vi "SeCrTs-RT_Main.vi"() -> ()   [LabVIEW 2022 SP3]
uses:
  <vilib>/Platform/TimedLoop/XDataNode/timing_clust.ctl
  <vilib>/Platform/TimedLoop/XDataNode/nitl_modes.ctl
  <vilib>/Platform/TimedLoop/XDataNode/wakeup.ctl
  RT Support/SeCrTs-RT_Global_R.vi
  <vilib>/platform/TimedLoop/XDataNode/XDataNode.xnode
  <vilib>/Platform/TimedLoop/XDataNode/XDNodeRunTimeDep.lvlib
panel:
  out "CDT":dbl
  # "RT main"
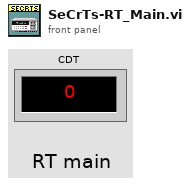
[diagram p1: front panel]
types:
  T1 = enum16{"Init", "Read 'All'", "Read 'n'", "Read '1'", "Write '1'", "Write 'n'", "Write 'All'"}
  T2 = cluster{"Device List":cluster{"AO Cards":tag[], "AI Cards":tag[], "DI Cards":tag[], "DO Cards":tag[]}, "Channel List":cluster{"AI Channel list":tag[], "AO Channel list":tag[], "DO Channel list ":tag[], "DI Channel list":tag[]}}
  T3 = cluster{"Drive Control":cluster{"En_Drive_A":bool, "En_Drive_L":bool, "Exit_Drive_A":bool, "Exit_Drive_L":bool}, "Drive_ATF Control":cluster{"S.Freq":dbl, "Ramp up Time":dbl, "Ramp down Time":dbl, "Drive Speed":dbl, "Drive condition":dbl}, "Drive_LOX Control":cluster{"S.Freq":dbl, "Ramp up Time":dbl, "Ramp down Time":dbl, "Drive Speed":dbl, "Drive condition":dbl}, "Aconnection ID":refnum<k5>, "Lconnection ID":refnum<k5>, "Loop Control":cluster{"Start DAQ":bool, "Stop DAQ":bool, "RT Stop":bool, "RT Exit":bool, "Start Seq":bool}}
  T4 = cluster{"AO Cards":tag[], "AI Cards":tag[], "DI Cards":tag[], "DO Cards":tag[]}
  T5 = cluster{"AI Channel list":tag[], "AO Channel list":tag[], "DO Channel list ":tag[], "DI Channel list":tag[]}
  T6 = typedef "SeCrTs-Data FIFO.ctl" = cluster{"Control":cluster{"AI_V_Data":refnum<queue>, "AI_C_Data":refnum<queue>, "AO_Data":refnum<queue>, "DO_Data":refnum<queue>, "DI_Data":refnum<queue>, "ACC_Data":refnum<queue>, "TC_Data":refnum<queue>, "Drive_A_C":refnum<queue>, "Drive_A_D":refnum<queue>, "Drive_L_C":refnum<queue>, "Drive_L_D":refnum<queue>}, "Display":cluster{"AI_V_Data D":refnum<queue>, "AI_C_Data D":refnum<queue>, "AO_Data D":refnum<queue>, "DO_Data D":refnum<queue>, "DI_Data D":refnum<queue>, "ACC_Data D":refnum<queue>, "TC_Data D":refnum<queue>, "Drive_A_C D":refnum<queue>, "Drive_A_D D":refnum<queue>, "Drive_L_C D":refnum<queue>, "Drive_L_D D":refnum<queue>}, "RD":cluster{"AI_V_Data RD":refnum<queue>, "AI_C_Data RD":refnum<queue>, "AO_Data RD":refnum<queue>, "DO_Data RD":refnum<queue>, "DI_Data RD":refnum<queue>, "ACC_Data RD":refnum<queue>, "TC_Data RD":refnum<queue>, "Drive_A_C RD":refnum<queue>, "Drive_A_D RD":refnum<queue>, "Drive_L_C RD":refnum<queue>, "Drive_L_D RD":refnum<queue>}}
  T7 = typedef "XDNodeRunTimeDep.lvlib/timing_clust.ctl" = cluster{"Expected End [f-1]":u64, "Actual End [f-1]":u64, "Finished Late? [f-1]":bool, "Expected End [i-1]":u64, "Actual End [i-1]":u64, "Finished Late? [i-1]":bool, "Expected Start [i]":u64, "Actual Start [i]":u64, "Expected Start [f]":u64, "Actual Start [f]":u64, "Source Name":string, "Structure Name":string, "Period":i64, "Deadline":i64, "Offset":i64, "Start":i64, "Priority":i32, "Timeout":i32, "Mode":T8, "Wakeup Reason":T9, "Error":errorcluster, "Source Type":string, "Secondary Source Type":string, "Global End Time":u64, "Global Start Time":u64, "Frame Duration":u64, "Iteration Duration":u64, "Assigned CPU":i32, "I/O Scan Engine Mode":u32}
  T8 = typedef "XDNodeRunTimeDep.lvlib/nitl_modes.ctl" = enum32{"No Change", "Process missed periods, maintain original phase", "Discard missed periods, maintain original phase", "Process missed periods, ignore original phase", "Discard missed periods, ignore original phase"}
  T9 = typedef "XDNodeRunTimeDep.lvlib/wakeup.ctl" = enum32{"Normal", "Aborted", "Asynchronous wakeup", "Timing source error", "Timed loop error", "Timeout"}
  T10 = cluster{cluster{"Sr. No.":string, "Time CDT":string, "Component ID":string, "Data Type":string, "Condition":string, "Range/Position":string, "No of Samples for Pass":string, "Event Duration":string, "Continuous /Cumulative":string, "Expected Delay":string, "Failure case Seq":string, "Current Sequence":string}[]}[]
  T11 = cluster{"AO config":cluster{"Channel_Name":string, "Channel_Number":string, "Default_Value":dbl, "Units":string}[], "AI config":cluster{"Channel_Name":string, "Channel_Number":string, "Pre_Scale_min":dbl, "Pre_Scale_max":dbl, "Sensor_min":dbl, "Sensor_max":dbl, "Units":string}[], "DI config":cluster{"Channel_Name":string, "Channel_Number":string, "Default_Value":bool, "DI invert?":bool}[], "DO config":cluster{"Channel_Name":string, "Channel_Number":string, "Default_Value":bool, "DO invert?":bool}[], "TC config":cluster{"Channel_Name":string, "Channel_Number":string, "Pre_Scale_min":dbl, "Pre_Scale_max":dbl, "units":i32, " type":i32}[], "ACC config":cluster{"Channel_Name":string, "Channel_Number":string, "Pre_Scale_min":dbl, "Pre_Scale_max":dbl, "Terminal configuration":i32, "Sensitivity":dbl, "Sensitivity units":i32}[], "SG config":cluster{"Channel_Name":string, "Channel_Number":string, "Pre_Scale_min":dbl, "Pre_Scale_max":dbl}[], "Strain Gauge Settings":cluster{"poisson ratio":dbl, "nominal gage resistance":dbl, "gage factor":dbl}, "Bridge Settings":cluster{"voltage excitation value":dbl, "voltage excitation source":i32, "initial bridge voltage":dbl, "lead wire resistance":dbl, "strain configuration":i32}, "Sample Rate":cluster{"AI Sample Rate":dbl[], "AO Sample Rate":dbl[], "DI Sample Rate":dbl[], "TC Sample Rate":dbl[], "DO Sample Rate":dbl[], "SG Sample Rate":dbl[], "ACC Sample Rate":dbl[]}}
  T12 = enum16{"Init", "Read", "Write 'All'", "Write 'n'", "Write Safe Value", "Write Start Time", "Overwrite Pattern", "Overwrite Pattern with Start", "Append Pattern", "Start Pattern Mode", "Abort Pattern Mode", "Read 1"}
  T13 = cluster{"S.Freq":dbl, "Ramp up Time":dbl, "Ramp down Time":dbl, "Drive Speed":dbl, "Drive condition":dbl}
  T14 = cluster{"Start DAQ":bool, "Stop DAQ":bool, "RT Stop":bool, "RT Exit":bool, "Start Seq":bool}
  T15 = cluster{"En_Drive_A":bool, "En_Drive_L":bool, "Exit_Drive_A":bool, "Exit_Drive_L":bool}
  T16 = cluster{"Manual HOLD":bool, "Automatic Hold AI":bool, "Abort":bool, "Automatic Hold DI":bool}
  T17 = cluster{"Channel_Name":string, "Channel_Number":string, "Default_Value":bool, "DO invert?":bool}[]
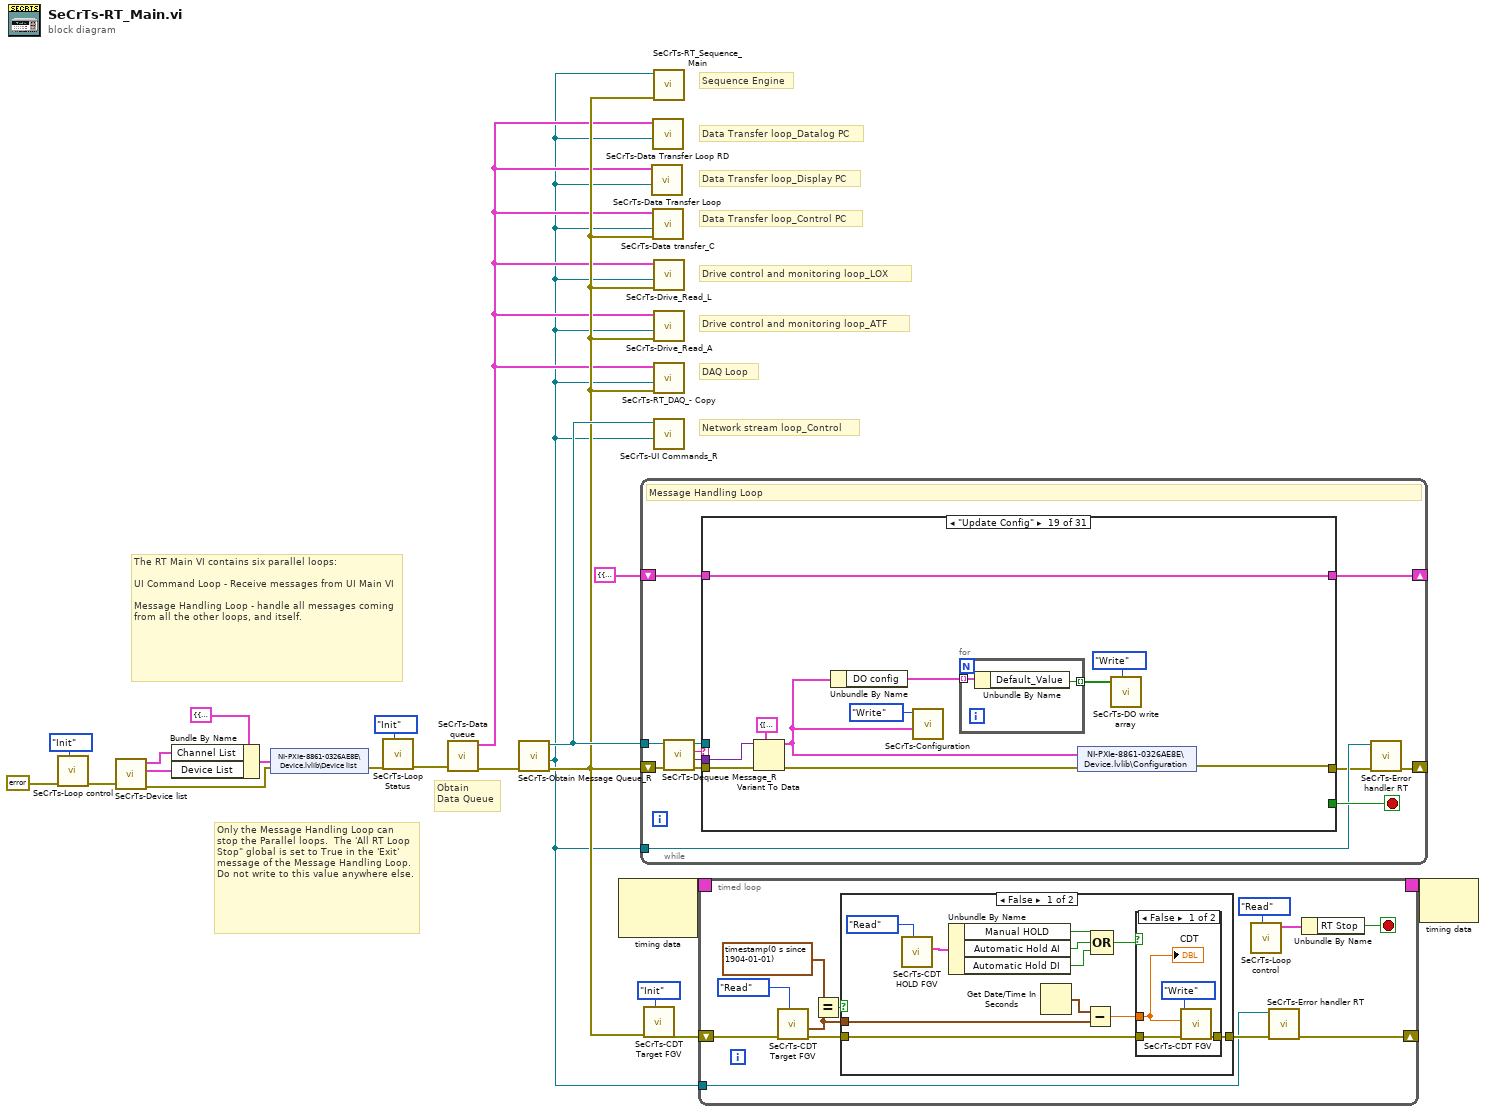
[diagram p0: block diagram]
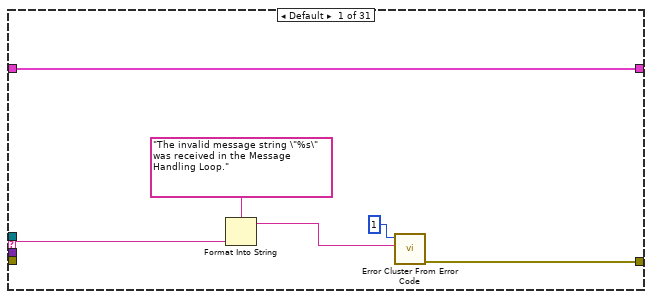
[diagram p4: hidden frame]
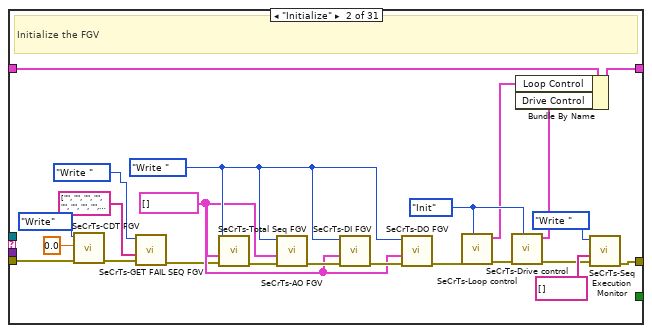
[diagram p5: hidden frame]
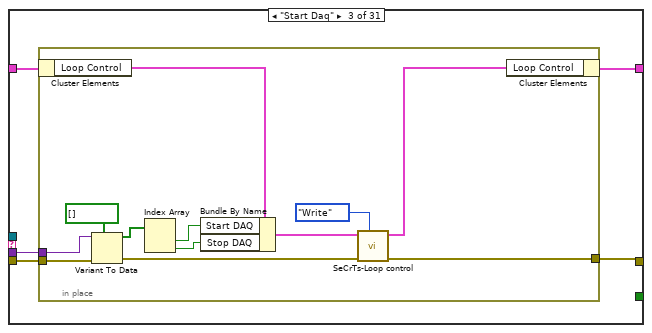
[diagram p6: hidden frame]
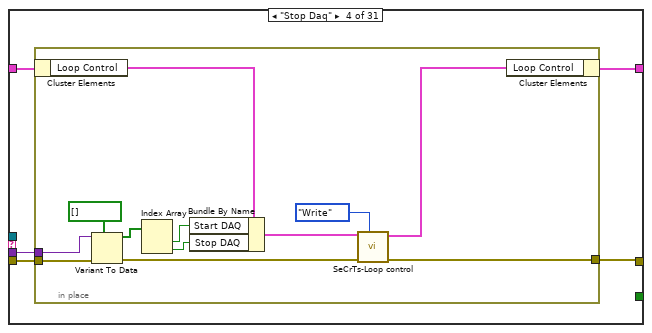
[diagram p7: hidden frame]
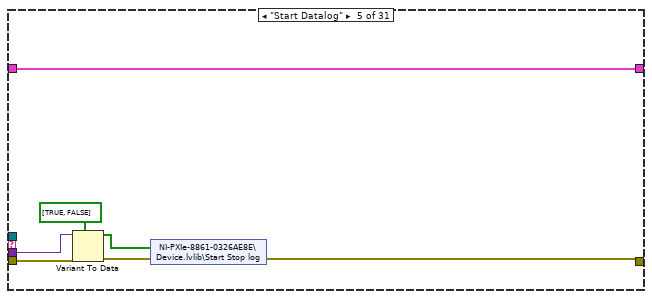
[diagram p8: hidden frame]
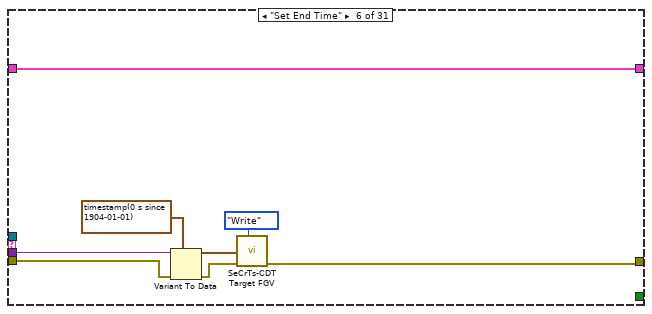
[diagram p9: hidden frame]
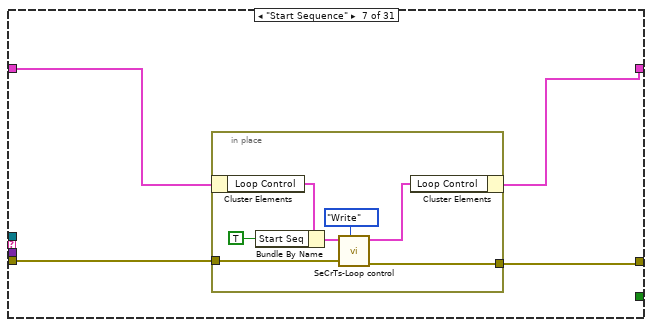
[diagram p10: hidden frame]
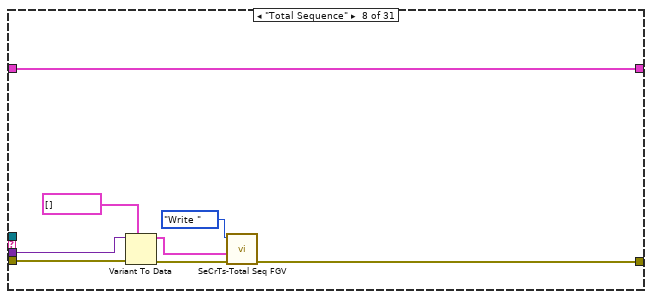
[diagram p11: hidden frame]
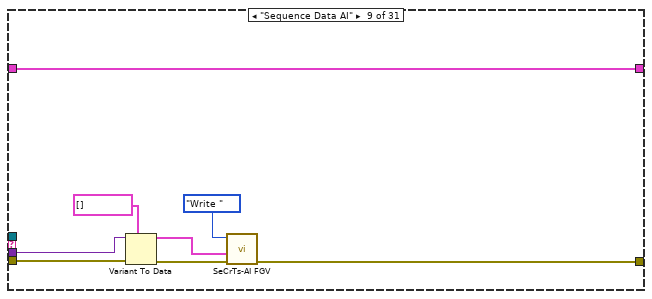
[diagram p12: hidden frame]
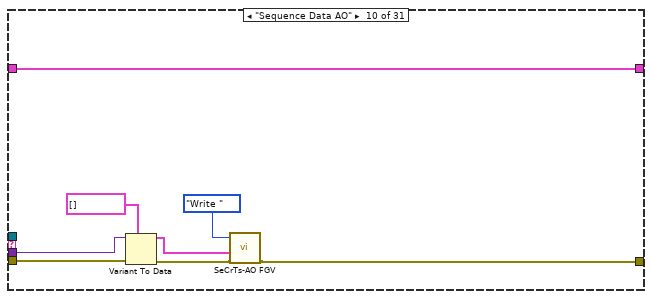
[diagram p13: hidden frame]
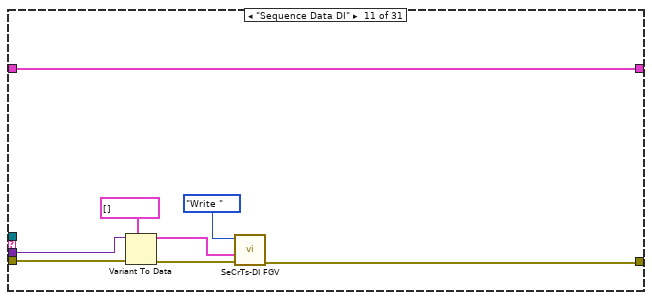
[diagram p14: hidden frame]
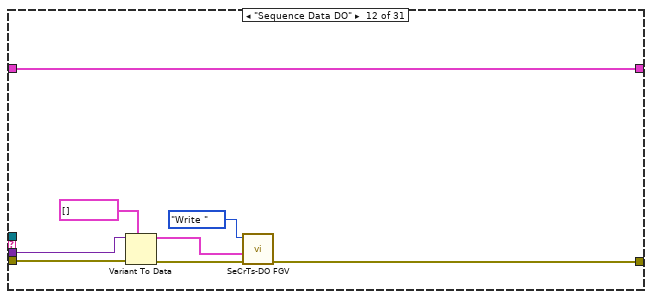
[diagram p15: hidden frame]
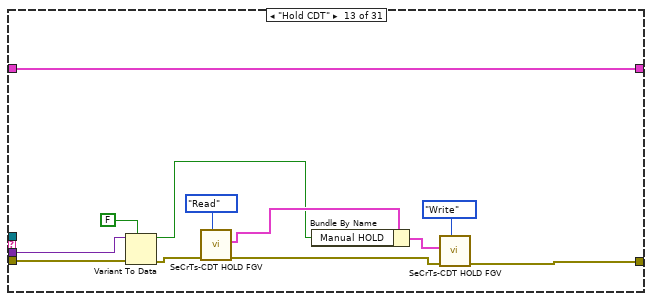
[diagram p16: hidden frame]
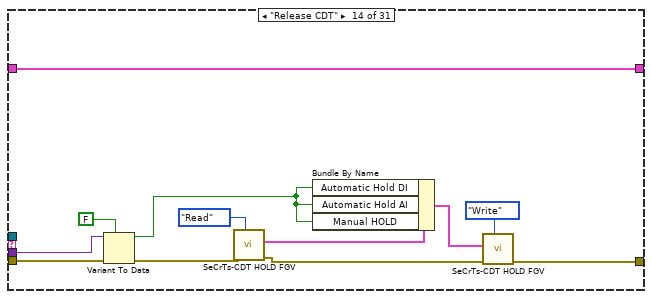
[diagram p17: hidden frame]
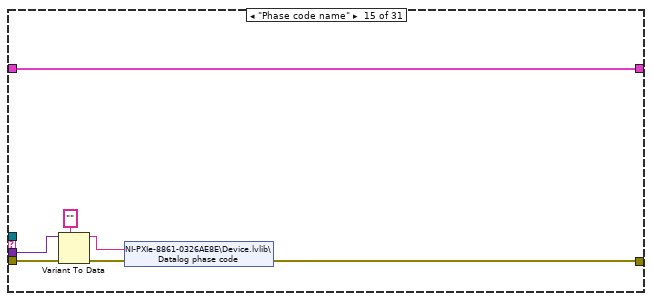
[diagram p18: hidden frame]
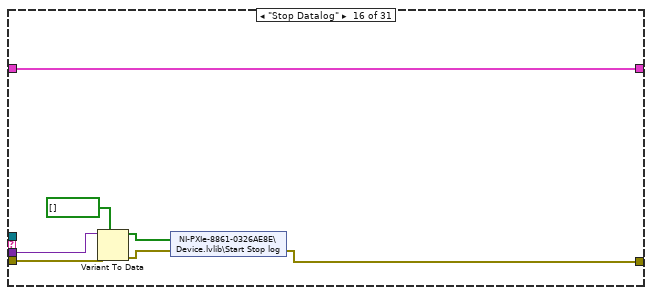
[diagram p19: hidden frame]
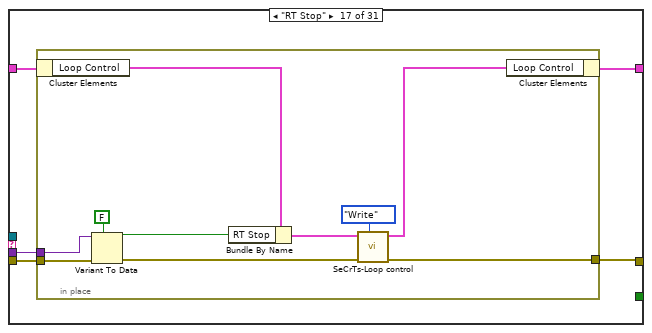
[diagram p20: hidden frame]
diagram:
  # "Sequence Engine"
  # "Data Transfer loop_Display PC"
  # "Data Transfer loop_Control PC"
  # "Drive control and monitoring loop_LOX"
  # "Drive control and monitoring loop_ATF"
  # "DAQ Loop"
  # "Data Transfer loop_Datalog PC"
  # "Obtain\nData Queue"
  # "Network stream loop_Control"
  # "The RT Main VI contains six parallel loops:\n\nUI Command Loop - Receive messages from UI Main VI\n\nMessage Handling Loop - handle all messages coming from all the other loops, and itself."
  # "Only the Message Handling Loop can stop the Parallel loops.  The 'All RT Loop Stop\" global is set to True in the 'Exit' message of the Message Handling Loop.  Do not write to this value anywhere else."
  n1 = call "SeCrTs-Loop control.vi"("Action"=enum16{"Init", "Write", "Read"}."Init", "error in (no error)"=errorcluster {"status"=FALSE, "code"=0, "source"=""} ("error constant")) -> ("error Out"=w6:errorcluster)  [unwired: 8 in, 1 out]
  n2 = call "SeCrTs-Device list.vi"("error in (no error)"=w6) -> ("error out"=w12:errorcluster, "Device List"=w14:T4, "Channel List"=w15:T5)  [unwired: 8 in]
  n3 = Bundle By Name(cluster=T2 {"Device List"={"AO Cards"=[], "AI Cards"=[], "DI Cards"=[], "DO Cards"=[]}, "Channel List"={"AI Channel list"=[], "AO Channel list"=[], "DO Channel list "=[], "DI Channel list"=[]}}, "Channel List"=w15, "Device List"=w14) -> (w13:T2)
  n4 = shared-variable "NI-PXIe-8861-0326AE8E\\Device.lvlib\\Device list"(w13, error in=w12) -> (error out=w10:errorcluster)
  n5 = call "SeCrTs-Loop Status.vi"("Option"=T1."Init", "error in (no error)"=w10) -> ("error out"=w9:errorcluster)  [unwired: 7 in, 2 out]
  n6 = call "SeCrTs-Data queue.vi"("error in"=w9) -> ("Data FIFO Ref"=w17:T6, "error out"=w18:errorcluster)  [unwired: 8 in]
  n7 = call "SeCrTs-Obtain Message Queue_R.vi"("error in (no error)"=w18) -> ("error out"=w20:errorcluster, "queue out"=w5:refnum<queue>, "Message Queue"=w21:refnum<queue>)  [unwired: 8 in]
  n8 = node-c288() -> (w4:T7)  [unwired: 2 in]
  n9 = while {
    shift-right: [w22] -> _
    shift-left: w20 -> [w33]
    tunnel: w21 -> [w31]
    shift-right: [w25] -> _
    shift-left: T3 {"Drive Control"={"En_Drive_A"=FALSE, "En_Drive_L"=FALSE, "Exit_Drive_A"=FALSE, "Exit_Drive_L"=FALSE}, "Drive_ATF Control"={"S.Freq"=0.0, "Ramp up Time"=0.0, "Ramp down Time"=0.0, "Drive Speed"=0.0, "Drive condition"=0.0}, "Drive_LOX Control"={"S.Freq"=0.0, "Ramp up Time"=0.0, "Ramp down Time"=0.0, "Drive Speed"=0.0, "Drive condition"=0.0}, "Aconnection ID"=refnum, "Lconnection ID"=refnum, "Loop Control"={"Start DAQ"=FALSE, "Stop DAQ"=FALSE, "RT Stop"=FALSE, "RT Exit"=FALSE, "Start Seq"=FALSE}} -> [w26]
    tunnel: w5 -> [w24]
    stop <- w27 stop-if-true
    # "Message Handling Loop"
    n10 = call "SeCrTs-Dequeue Message_R.vi"("error in (no error)"=w33, "Message Queue"=w31) -> ("error out"=w29:errorcluster, "Message Data"=w30:variant, "Message"=w32:string, "dup Message Queue"=w28:refnum<queue>)  [unwired: 6 in]
    n11 = case shown="\"Update Config\"" w32 {
      selector: w32 -> [w35 _ _ _ _ _ _ _ _ _ _ _ _ _ _ _ _ _ _ _ _ _ _ _ _ _ _ _ _ _ _]
      tunnel: w28 -> [_ _ _ _ _ _ _ _ _ _ _ _ _ _ _ _ _ _ _ _ _ _ _ _ _ _ _ _ _ _ w365]
      tunnel: w30 -> [_ _ w65 w82 w101 w110 _ w126 w134 w144 w152 w160 w172 w181 w191 w196 w203 _ w224 _ w246 _ w253 w267 w282 w297 w312 w336 _ _ w363]
      tunnel: w29 -> [_ w55 w67 w84 w102 w109 w113 w128 w136 w145 w153 w161 w173 w184 w192 w197 w205 _ w225 w231 w247 _ w254 w268 w283 w298 w313 w337 _ _ w364]
      tunnel: [w34 w41 w66 w83 w97 w105 w114 w124 w133 w142 w150 w159 w169 w183 w187 w194 w204 _ w217 w230 w243 _ w252 w266 w281 w296 w311 w335 _ _ w362] -> w23
      tunnel: [_ _ _ _ _ _ _ _ _ _ _ _ _ _ _ _ _ _ _ _ _ _ _ _ _ _ _ _ _ _ w361] -> w27
      tunnel: w26 -> [w39 w58 w64 w81 w103 w111 w115 w130 w138 w146 w154 w162 w174 w186 w193 w200 w202 w216 w227 w233 w248 w249 w251 w265 w280 w295 w310 w334 w357 w358 w360]
      tunnel: [w39 w57 w63 w80 w103 w111 w112 w130 w138 w146 w154 w162 w174 w186 w193 w200 w201 w216 w227 w232 w248 w249 w250 _ w279 w294 w309 w333 w357 w358 w359] -> w25
      frame Default {
        n12 = Format Into String(format string="The invalid message string \"%s\" was received in the Message Handling Loop." ("Unknown Message Error Text"), w35) -> (resulting string=w36:string)  [unwired: 2 in, 1 out]
        n13 = call <vilib>:"Error Cluster From Error Code.vi"("error message (\"\")"=w36, "error code (0)"=1) -> ("error out"=w34:errorcluster)  [unwired: 7 in]
      }
      frame "Initialize" {
        w48 = T10 [] ("Array")
        w56 = enum16{"Read", "Write "}."Write " ("Enum")
        w61 = enum16{"Init", "Write", "Read"}."Init" ("Action")
        # "Initialize the FGV"
        n14 = call "SeCrTs-CDT FGV.vi"("error in (no error)"=w55, "CDT"=0.0, "Write/Read"=enum16{"Write", "Read"}."Write") -> ("error Out"=w43:errorcluster)  [unwired: 7 in, 1 out]
        n15 = call "SeCrTs-GET FAIL SEQ FGV.vi"("error in"=w43, "Failure \ncase Seq"=string[] ["", "", "", "", "", "", "", "", "", ""] ("Failure \ncase Seq"), "Enum"=enum16{"Read", "Write "}."Write ") -> ("error out"=w42:errorcluster)  [unwired: 7 in, 1 out]
        n16 = call "SeCrTs-Total Seq FGV.vi"("error in"=w42, "Total Seq  IN"=w48, "Enum"=w56) -> ("error out"=w54:errorcluster)  [unwired: 7 in, 1 out]
        n17 = call "SeCrTs-AO FGV.vi"("error in"=w54, "AO Seq  IN"=w48, "Enum"=w56) -> ("error out"=w53:errorcluster)  [unwired: 7 in, 1 out]
        n18 = call "SeCrTs-DI FGV.vi"("error in"=w53, "DI Seq  IN"=w48, "Enum"=w56) -> ("error out"=w52:errorcluster)  [unwired: 7 in, 1 out]
        n19 = call "SeCrTs-DO FGV.vi"("error in"=w52, "DO Seq  IN"=w48, "Enum"=w56) -> ("error out"=w51:errorcluster)  [unwired: 7 in, 1 out]
        n20 = call "SeCrTs-Loop control.vi"("Action"=w61, "error in (no error)"=w51) -> ("error Out"=w62:errorcluster, "Loop Control out"=w60:T14)  [unwired: 8 in]
        n21 = call "SeCrTs-Drive control.vi"("Action"=w61, "error in"=w62) -> ("error Out"=w40:errorcluster, "Loop Control Out"=w59:T15)  [unwired: 8 in]
        n22 = Bundle By Name(cluster=w58, "Loop Control"=w60, "Drive Control"=w59) -> (w57:T3)
        n23 = call "SeCrTs-Seq Execution Monitor.vi"("error in"=w40, "Seq Monitor"=string[] [], "Enum"=enum16{"Read", "Write "}."Write ") -> ("error out"=w41:errorcluster)  [unwired: 7 in, 1 out]
      }
      frame "Start Daq" {
        n24 = in-place {
          in-place-border: w67 -> [w78]
          in-place-border: [w75] -> w66
          in-place-border: w65 -> [w74]
          n25 = in-place-cluster #1(w64) -> ("Loop Control"=w73:T14)
          n26 = Variant To Data(error in=w78, type=bool[] [], Variant=w74) -> (data=w70:bool[], error out=w76:errorcluster)
          n27 = Index Array(array=w70) -> (element #1=w69:bool, element #2=w68:bool)  [unwired: 2 in]
          n28 = Bundle By Name(cluster=w73, "Start DAQ"=w69, "Stop DAQ"=w68) -> (w72:T14)
          n29 = call "SeCrTs-Loop control.vi"("Action"=enum16{"Init", "Write", "Read"}."Write", "error in (no error)"=w76, "Loop Control In"=w72) -> ("error Out"=w75:errorcluster, "Loop Control out"=w71:T14)  [unwired: 7 in]
          n30 = in-place-cluster #1("Loop Control"=w71) -> (w63:T3)
        }
      }
      frame "Stop Daq" {
        n31 = in-place {
          in-place-border: w84 -> [w95]
          in-place-border: [w92] -> w83
          in-place-border: w82 -> [w91]
          n32 = in-place-cluster #2(w81) -> ("Loop Control"=w90:T14)
          n33 = Variant To Data(error in=w95, type=bool[] [], Variant=w91) -> (data=w87:bool[], error out=w93:errorcluster)
          n34 = Index Array(array=w87) -> (element #1=w86:bool, element #2=w85:bool)  [unwired: 2 in]
          n35 = Bundle By Name(cluster=w90, "Start DAQ"=w86, "Stop DAQ"=w85) -> (w89:T14)
          n36 = call "SeCrTs-Loop control.vi"("Action"=enum16{"Init", "Write", "Read"}."Write", "error in (no error)"=w93, "Loop Control In"=w89) -> ("error Out"=w92:errorcluster, "Loop Control out"=w88:T14)  [unwired: 7 in]
          n37 = in-place-cluster #2("Loop Control"=w88) -> (w80:T3)
        }
      }
      frame "Start Datalog" {
        n38 = Variant To Data(error in=w102, type=bool[] [TRUE, FALSE] ("Start Stop log"), Variant=w101) -> (data=w99:bool[], error out=w98:errorcluster)
        n39 = shared-variable "NI-PXIe-8861-0326AE8E\\Device.lvlib\\Start Stop log"(w99, error in=w98) -> (error out=w97:errorcluster)
      }
      frame "Set End Time" {
        n40 = Variant To Data(error in=w109, type=timestamp(0 s since 1904-01-01) ("current time"), Variant=w110) -> (data=w107:timestamp, error out=w106:errorcluster)
        n41 = call "SeCrTs-CDT Target FGV.vi"("Enum"=enum16{"Write", "Read", "Init"}."Write", "error in"=w106, "Time Stamp"=w107) -> ("error out"=w105:errorcluster)  [unwired: 7 in, 1 out]
      }
      frame "Start Sequence" {
        n42 = in-place {
          in-place-border: w113 -> [w117]
          in-place-border: [w116] -> w114
          n43 = in-place-cluster #3(w115) -> ("Loop Control"=w122:T14)
          n44 = Bundle By Name(cluster=w122, "Start Seq"=TRUE ("Start DAQ")) -> (w119:T14)
          n45 = call "SeCrTs-Loop control.vi"("Action"=enum16{"Init", "Write", "Read"}."Write", "error in (no error)"=w117, "Loop Control In"=w119) -> ("error Out"=w116:errorcluster, "Loop Control out"=w118:T14)  [unwired: 7 in]
          n46 = in-place-cluster #3("Loop Control"=w118) -> (w112:T3)
        }
      }
      frame "Total Sequence" {
        n47 = Variant To Data(error in=w128, type=T10 [] ("Array"), Variant=w126) -> (data=w125:T10, error out=w127:errorcluster)
        n48 = call "SeCrTs-Total Seq FGV.vi"("error in"=w127, "Total Seq  IN"=w125, "Enum"=enum16{"Read", "Write "}."Write ") -> ("error out"=w124:errorcluster)  [unwired: 7 in, 1 out]
      }
      frame "Sequence Data AI" {
        n49 = Variant To Data(error in=w136, type=T10 [] ("Array"), Variant=w134) -> (data=w132:T10, error out=w135:errorcluster)
        n50 = call "SeCrTs-AI FGV.vi"("error in"=w135, "AI Seq  IN"=w132, "Enum"=enum16{"Read", "Write "}."Write ") -> ("error out"=w133:errorcluster)  [unwired: 7 in, 1 out]
      }
      frame "Sequence Data AO" {
        n51 = Variant To Data(error in=w145, type=T10 [] ("Array"), Variant=w144) -> (data=w141:T10, error out=w143:errorcluster)
        n52 = call "SeCrTs-AO FGV.vi"("error in"=w143, "AO Seq  IN"=w141, "Enum"=enum16{"Read", "Write "}."Write ") -> ("error out"=w142:errorcluster)  [unwired: 7 in, 1 out]
      }
      frame "Sequence Data DI" {
        n53 = Variant To Data(error in=w153, type=T10 [] ("Array"), Variant=w152) -> (data=w147:T10, error out=w151:errorcluster)
        n54 = call "SeCrTs-DI FGV.vi"("error in"=w151, "DI Seq  IN"=w147, "Enum"=enum16{"Read", "Write "}."Write ") -> ("error out"=w150:errorcluster)  [unwired: 7 in, 1 out]
      }
      frame "Sequence Data DO" {
        n55 = Variant To Data(error in=w161, type=T10 [] ("Array"), Variant=w160) -> (data=w155:T10, error out=w158:errorcluster)
        n56 = call "SeCrTs-DO FGV.vi"("error in"=w158, "DO Seq  IN"=w155, "Enum"=enum16{"Read", "Write "}."Write ") -> ("error out"=w159:errorcluster)  [unwired: 7 in, 1 out]
      }
      frame "Hold CDT" {
        n57 = Variant To Data(error in=w173, type=FALSE, Variant=w172) -> (data=w163:bool, error out=w167:errorcluster)
        n58 = call "SeCrTs-CDT HOLD FGV.vi"("Write/Read"=enum16{"Write", "Read"}."Read", "error in (no error)"=w167) -> ("error Out"=w166:errorcluster, "HOLD and Abort Out"=w164:T16)  [unwired: 6 in]
        n59 = Bundle By Name(cluster=w164, "Manual HOLD"=w163) -> (w165:T16)
        n60 = call "SeCrTs-CDT HOLD FGV.vi"("Write/Read"=enum16{"Write", "Read"}."Write", "error in (no error)"=w166, "HOLD and Abort"=w165) -> ("error Out"=w169:errorcluster)  [unwired: 5 in, 1 out]
      }
      frame "Release CDT" {
        n61 = Variant To Data(error in=w184, type=FALSE, Variant=w181) -> (data=w176:bool, error out=w175:errorcluster)
        n62 = call "SeCrTs-CDT HOLD FGV.vi"("Write/Read"=enum16{"Write", "Read"}."Read", "error in (no error)"=w175) -> ("error Out"=w178:errorcluster, "HOLD and Abort Out"=w179:T16)  [unwired: 6 in]
        n63 = Bundle By Name(cluster=w179, "Automatic Hold DI"=w176, "Automatic Hold AI"=w176, "Manual HOLD"=w176) -> (w177:T16)
        n64 = call "SeCrTs-CDT HOLD FGV.vi"("Write/Read"=enum16{"Write", "Read"}."Write", "error in (no error)"=w178, "HOLD and Abort"=w177) -> ("error Out"=w183:errorcluster)  [unwired: 5 in, 1 out]
      }
      frame "Phase code name" {
        n65 = Variant To Data(error in=w192, type="" ("Datalog phase code"), Variant=w191) -> (data=w188:string, error out=w189:errorcluster)
        n66 = shared-variable "NI-PXIe-8861-0326AE8E\\Device.lvlib\\Datalog phase code"(w188, error in=w189) -> (error out=w187:errorcluster)
      }
      frame "Stop Datalog" {
        n67 = Variant To Data(error in=w197, type=bool[] [], Variant=w196) -> (data=w199:bool[], error out=w198:errorcluster)
        n68 = shared-variable "NI-PXIe-8861-0326AE8E\\Device.lvlib\\Start Stop log"(w199, error in=w198) -> (error out=w194:errorcluster)
      }
      frame "RT Stop" {
        n69 = in-place {
          in-place-border: w205 -> [w214]
          in-place-border: [w210] -> w204
          in-place-border: w203 -> [w209]
          n70 = in-place-cluster #4(w202) -> ("Loop Control"=w208:T14)
          n71 = Variant To Data(error in=w214, type=FALSE, Variant=w209) -> (data=w213:bool, error out=w211:errorcluster)
          n72 = Bundle By Name(cluster=w208, "RT Stop"=w213) -> (w206:T14)
          n73 = call "SeCrTs-Loop control.vi"("Action"=enum16{"Init", "Write", "Read"}."Write", "error in (no error)"=w211, "Loop Control In"=w206) -> ("error Out"=w210:errorcluster, "Loop Control out"=w207:T14)  [unwired: 7 in]
          n74 = in-place-cluster #4("Loop Control"=w207) -> (w201:T3)
        }
      }
      frame "IP Config" {
      }
      frame "Update Config" {
        n75 = Variant To Data(error in=w225, type=T11 {"AO config"=[], "AI config"=[], "DI config"=[], "DO config"=[], "TC config"=[{"Channel_Name"="", "Channel_Number"="", "Pre_Scale_min"=0.0, "Pre_Scale_max"=0.0, "units"=4, " type"=7}], "ACC config"=[], "SG config"=[], "Strain Gauge Settings"={"poisson ratio"=0.3, "nominal gage resistance"=120.0, "gage factor"=2.08}, "Bridge Settings"={"voltage excitation value"=3.3, "voltage excitation source"=10200, "initial bridge voltage"=0.0, "lead wire resistance"=1.7, "strain configuration"=10271}, "Sample Rate"={"AI Sample Rate"=[], "AO Sample Rate"=[], "DI Sample Rate"=[], "TC Sample Rate"=[], "DO Sample Rate"=[], "SG Sample Rate"=[], "ACC Sample Rate"=[]}} ("Config in"), Variant=w224) -> (data=w221:T11, error out=w218:errorcluster)
        n76 = Unbundle By Name(w221) -> ("DO config"=w220:T17)
        n77 = call "SeCrTs-Configuration.vi"("Config in"=w221, "Enum"=enum16{"Write", "Read"}."Write") -> ()  [unwired: 9 in, 1 out]
        n78 = for {
          tunnel: w220 -> [w229] mode=indexing
          tunnel: [w228] -> w219 mode=indexing
          n79 = Unbundle By Name(w229) -> ("Default_Value"=w228:bool)
        }
        n80 = shared-variable "NI-PXIe-8861-0326AE8E\\Device.lvlib\\Configuration"(w221, error in=w218) -> (error out=w217:errorcluster)
        n81 = call "SeCrTs-DO write array.vi"("Enum"=enum16{"Write", "Read"}."Write", "DO Array"=w219) -> ()  [unwired: 9 in, 1 out]
      }
      frame "Revert Sequence" {
        n82 = in-place {
          in-place-border: w231 -> [w235]
          in-place-border: [w234] -> w230
          n83 = in-place-cluster #5(w233) -> ("Loop Control"=w240:T14)
          n84 = Bundle By Name(cluster=w240, "Start Seq"=FALSE ("Start DAQ")) -> (w237:T14)
          n85 = call "SeCrTs-Loop control.vi"("Action"=enum16{"Init", "Write", "Read"}."Write", "error in (no error)"=w235, "Loop Control In"=w237) -> ("error Out"=w234:errorcluster, "Loop Control out"=w236:T14)  [unwired: 7 in]
          n86 = in-place-cluster #5("Loop Control"=w236) -> (w232:T3)
        }
      }
      frame "Write DO" {
        n87 = Variant To Data(error in=w247, type=bool[] [] ("DO Array"), Variant=w246) -> (data=w242:bool[], error out=w244:errorcluster)
        n88 = call "SeCrTs-DO Data FGV.vi"("DO Values In"=w242, "Option"=T12."Write 'All'", "error in (no error)"=w244) -> ("error out"=w243:errorcluster)  [unwired: 6 in, 6 out]
      }
      frame "Update Valve State" {
      }
      frame "Connect Drive ATF" {
        n89 = in-place {
          in-place-border: w254 -> [w263]
          in-place-border: w253 -> [w262]
          in-place-border: [w258] -> w252
          n90 = in-place-cluster #6(w251) -> ("Drive Control"=w257:T15)
          n91 = Variant To Data(error in=w263, type=FALSE, Variant=w262) -> (data=w261:bool, error out=w259:errorcluster)
          n92 = Bundle By Name(cluster=w257, "En_Drive_A"=w261) -> (w256:T15)
          n93 = call "SeCrTs-Drive control.vi"("Action"=enum16{"Init", "Write", "Read"}."Write", "error in"=w259, "Loop Control In"=w256) -> ("error Out"=w258:errorcluster, "Loop Control Out"=w255:T15)  [unwired: 7 in]
          n94 = in-place-cluster #6("Drive Control"=w255) -> (w250:T3)
        }
      }
      frame "Exit Drive ATF" {
        n95 = in-place {
          in-place-border: w268 -> [w277]
          in-place-border: w267 -> [w276]
          in-place-border: [w271] -> w266
          n96 = in-place-cluster #7(w265) -> ("Drive Control"=w270:T15)
          n97 = Variant To Data(error in=w277, type=FALSE, Variant=w276) -> (data=w275:bool, error out=w272:errorcluster)
          n98 = Bundle By Name(cluster=w270, "Exit_Drive_A"=w275) -> (w274:T15)
          n99 = call "SeCrTs-Drive control.vi"("Action"=enum16{"Init", "Write", "Read"}."Write", "error in"=w272, "Loop Control In"=w274) -> ("error Out"=w271:errorcluster, "Loop Control Out"=w269:T15)  [unwired: 7 in]
          n100 = in-place-cluster #7("Drive Control"=w269) -> ()  [unwired: 1 out]
        }
      }
      frame "Exit Drive LOX" {
        n101 = in-place {
          in-place-border: w283 -> [w292]
          in-place-border: w282 -> [w291]
          in-place-border: [w287] -> w281
          n102 = in-place-cluster #8(w280) -> ("Drive Control"=w284:T15)
          n103 = Variant To Data(error in=w292, type=FALSE, Variant=w291) -> (data=w290:bool, error out=w288:errorcluster)
          n104 = Bundle By Name(cluster=w284, "Exit_Drive_L"=w290) -> (w285:T15)
          n105 = call "SeCrTs-Drive control.vi"("Action"=enum16{"Init", "Write", "Read"}."Write", "error in"=w288, "Loop Control In"=w285) -> ("error Out"=w287:errorcluster, "Loop Control Out"=w286:T15)  [unwired: 7 in]
          n106 = in-place-cluster #8("Drive Control"=w286) -> (w279:T3)
        }
      }
      frame "Connect Drive LOX" {
        n107 = in-place {
          in-place-border: w298 -> [w307]
          in-place-border: w297 -> [w306]
          in-place-border: [w302] -> w296
          n108 = in-place-cluster #9(w295) -> ("Drive Control"=w301:T15)
          n109 = Variant To Data(error in=w307, type=FALSE, Variant=w306) -> (data=w305:bool, error out=w303:errorcluster)
          n110 = Bundle By Name(cluster=w301, "En_Drive_L"=w305) -> (w299:T15)
          n111 = call "SeCrTs-Drive control.vi"("Action"=enum16{"Init", "Write", "Read"}."Write", "error in"=w303, "Loop Control In"=w299) -> ("error Out"=w302:errorcluster, "Loop Control Out"=w300:T15)  [unwired: 7 in]
          n112 = in-place-cluster #9("Drive Control"=w300) -> (w294:T3)
        }
      }
      frame "Update Drive ATF" {
        n113 = in-place {
          in-place-border: w313 -> [w324]
          in-place-border: w312 -> [w323]
          in-place-border: [w318] -> w311
          n114 = in-place-cluster #10(w310) -> ("Aconnection ID"=w315:refnum<k5>)
          n115 = Variant To Data(error in=w324, type=T13 {"S.Freq"=0.0, "Ramp up Time"=0.0, "Ramp down Time"=0.0, "Drive Speed"=0.0, "Drive condition"=0.0} ("Drive_ATF Control"), Variant=w323) -> (data=w322:T13, error out=w319:errorcluster)
          n116 = Cluster To Array(cluster=w322) -> (array=w321:dbl[])
          n117 = for {
            tunnel: w321 -> [w332] mode=indexing
            tunnel: i32[] [17, 18, 19, 20, 21] -> [w331] mode=indexing
            tunnel: [w330] -> w317 mode=indexing
            n118 = call "SeCrTs-Drive_Message.vi"("Input"=w332, "Packet \nIdentifier"=w331) -> ("String"=w330:string)  [unwired: 9 in]
          }
          n119 = for {
            tunnel: w317 -> [w327] mode=indexing
            shift-right: [w328] -> w318
            shift-left: w319 -> [w329]
            tunnel: w315 -> [w326]
            tunnel: [w325] -> w314
            n120 = TCP Write(connection ID=w326, data in=w327, error in (no error)=w329) -> (connection ID out=w325:refnum<k5>, error out=w328:errorcluster)  [unwired: 1 in, 1 out]
          }
          n121 = in-place-cluster #10("Aconnection ID"=w314) -> (w309:T3)
        }
      }
      frame "Update Drive LOX" {
        n122 = in-place {
          in-place-border: w337 -> [w348]
          in-place-border: w336 -> [w347]
          in-place-border: [w342] -> w335
          n123 = in-place-cluster #11(w334) -> ("Lconnection ID"=w339:refnum<k5>)
          n124 = Variant To Data(error in=w348, type=T13 {"S.Freq"=0.0, "Ramp up Time"=0.0, "Ramp down Time"=0.0, "Drive Speed"=0.0, "Drive condition"=0.0} ("Drive_ATF Control"), Variant=w347) -> (data=w346:T13, error out=w343:errorcluster)
          n125 = Cluster To Array(cluster=w346) -> (array=w345:dbl[])
          n126 = for {
            tunnel: w345 -> [w356] mode=indexing
            tunnel: i32[] [17, 18, 19, 20, 21] -> [w355] mode=indexing
            tunnel: [w354] -> w341 mode=indexing
            n127 = call "SeCrTs-Drive_Message.vi"("Input"=w356, "Packet \nIdentifier"=w355) -> ("String"=w354:string)  [unwired: 9 in]
          }
          n128 = for {
            tunnel: w341 -> [w351] mode=indexing
            shift-right: [w352] -> w342
            shift-left: w343 -> [w353]
            tunnel: w339 -> [w350]
            tunnel: [w349] -> w338
            n129 = TCP Write(connection ID=w350, data in=w351, error in (no error)=w353) -> (connection ID out=w349:refnum<k5>, error out=w352:errorcluster)  [unwired: 1 in, 1 out]
          }
          n130 = in-place-cluster #11("Lconnection ID"=w338) -> (w333:T3)
        }
      }
      frame "Phase Code Update" {
      }
      frame "Abort" {
      }
      frame "RT Exit" {
        # "Initialize- Currently a no-op for the RT Main VI"
        n131 = in-place {
          in-place-border: w365 -> [w388]
          in-place-border: w364 -> [w386]
          in-place-border: w363 -> [w384]
          in-place-border: [w380] -> w362
          in-place-border: [TRUE] -> w361
          w379 = enum16{"Init", "Write", "Read"}."Write" ("Action")
          n132 = in-place-cluster #12(w360) -> ("Loop Control"=w374:T14, "Drive Control"=w373:T15)
          n133 = Variant To Data(error in=w386, type=FALSE, Variant=w384) -> (data=w382:bool, error out=w385:errorcluster)
          n134 = Bundle By Name(cluster=w373, "Exit_Drive_A"=w382, "Exit_Drive_L"=w382) -> (w372:T15)
          n135 = Release Queue(queue=w388, error in (no error)=w385) -> (error out=w383:errorcluster)  [unwired: 1 in, 2 out]
          n136 = Bundle By Name(cluster=w374, "RT Exit"=w382) -> (w371:T14)
          n137 = call "SeCrTs-Loop control.vi"("Action"=w379, "error in (no error)"=w383, "Loop Control In"=w371) -> ("error Out"=w381:errorcluster, "Loop Control out"=w369:T14)  [unwired: 7 in]
          n138 = call "SeCrTs-Drive control.vi"("Action"=w379, "error in"=w381, "Loop Control In"=w372) -> ("error Out"=w380:errorcluster, "Loop Control Out"=w370:T15)  [unwired: 7 in]
          n139 = global read "SeCrTs-RT_Global_R.vi" "RT Writer Stream_DD"() -> (w366:refnum<k21>)
          n140 = global read "SeCrTs-RT_Global_R.vi" "RT Writer Stream_D"() -> (w367:refnum<k21>)
          n141 = global read "SeCrTs-RT_Global_R.vi" "RT Writer Stream_C"() -> (w368:refnum<k21>)
          n142 = global read "SeCrTs-RT_Global_R.vi" "UI Writer stream"() -> (w378:refnum<k21>)
          n143 = in-place-cluster #12("Loop Control"=w369, "Drive Control"=w370) -> (w359:T3)
          n144 = Flush Stream(11:w368) -> (0:w376:errorcluster, 3:w377:refnum<k21>)  [unwired: 3 in, 1 out]
          n145 = Destroy Stream Endpoint(11:w378) -> ()  [unwired: 1 in, 1 out]
          n146 = Destroy Stream Endpoint(8:w376, 11:w377) -> ()  [unwired: 1 out]
          n147 = Destroy Stream Endpoint(11:w367) -> ()  [unwired: 1 in, 1 out]
          n148 = Destroy Stream Endpoint(11:w366) -> ()  [unwired: 1 in, 1 out]
        }
      }
    }
    n149 = call "SeCrTs-Error handler RT.vi"("error in"=w23, "Message Queue"=w24) -> ("error out"=w22:errorcluster)  [unwired: 8 in, 1 out]
  }
  n150 = call "SeCrTs-CDT Target FGV.vi"("Enum"=enum16{"Write", "Read", "Init"}."Init", "error in"=w20) -> ("error out"=w2:errorcluster)  [unwired: 8 in, 1 out]
  n151 = call "SeCrTs-Data Transfer Loop.vi"("Message Queue 2"=w5, "Data FIFO Ref"=w17) -> ()  [unwired: 10 in]
  n152 = call "SeCrTs-Data Transfer Loop RD.vi"("Message Queue 2"=w5, "Data FIFO Ref"=w17) -> ()  [unwired: 10 in]
  n153 = call "SeCrTs-Data transfer_C.vi"("Data FIFO Ref"=w17, "Message Queue"=w5, "error constant"=w20) -> ()  [unwired: 7 in, 1 out]
  n154 = call "SeCrTs-RT_Sequence_Main.vi"("error in"=w20, "Message Queue"=w5) -> ()  [unwired: 9 in, 1 out]
  n155 = call "SeCrTs-Drive_Read_L.vi"("error in"=w20, "Message Queue"=w5, "Data FIFO Ref"=w17) -> ()  [unwired: 8 in, 1 out]
  n156 = call "SeCrTs-Drive_Read_A.vi"("error in"=w20, "Er"=w5, "Data FIFO Ref"=w17) -> ()  [unwired: 8 in, 1 out]
  n157 = call "SeCrTs-RT_DAQ_- Copy.vi"("error in"=w20, "er"=w5, "Data FIFO Ref"=w17) -> ()  [unwired: 8 in, 1 out]
  n158 = call "SeCrTs-UI Commands_R.vi"("Er"=w5, "Message Queue"=w21) -> ()  [unwired: 10 in]
  n159 = timed-loop {
    timing: w4 -> [_]
    timing-out: [_] -> w3
    shift-right: [w391] -> _
    shift-left: w2 -> [w396]
    tunnel: w5 -> [w390]
    stop <- w400 stop-if-true
    n160 = call "SeCrTs-CDT Target FGV.vi"("Enum"=enum16{"Write", "Read", "Init"}."Read", "error in"=w396) -> ("error out"=w395:errorcluster, "Time StampOut"=w397:timestamp)  [unwired: 8 in]
    n161 = Equal?(x=timestamp(0 s since 1904-01-01), y=w397) -> (x = y?=w399:bool)
    n162 = case shown="False" w399 {
      tunnel: w397 -> [w409 _]
      tunnel: w395 -> [w408 w417]
      tunnel: [w407 w417] -> w392
      frame False {
        n163 = call "SeCrTs-CDT HOLD FGV.vi"("Write/Read"=enum16{"Write", "Read"}."Read") -> ("HOLD and Abort Out"=w405:T16)  [unwired: 7 in, 1 out]
        n164 = Unbundle By Name(w405) -> ("Manual HOLD"=w404:bool, "Automatic Hold AI"=w403:bool, "Automatic Hold DI"=w402:bool)
        n165 = Get Date/Time In Seconds() -> (seconds since 1Jan1904=w411:timestamp)
        n166 = Subtract(x=w411, y=w409) -> (x-y=w410:dbl)
        n167 = Compound Arithmetic op=OR(w404, w403, w402) -> (w401:bool)
        n168 = case shown="False" w401 {
          tunnel: w410 -> [w414 _]
          tunnel: w408 -> [w413 w416]
          tunnel: [w412 w416] -> w407
          frame False {
            n169 = call "SeCrTs-CDT FGV.vi"("error in (no error)"=w413, "CDT"=w414, "Write/Read"=enum16{"Write", "Read"}."Write") -> ("error Out"=w412:errorcluster)  [unwired: 7 in, 1 out]
            "CDT" <- w414
          }
          frame True {
          }
        }
      }
      frame True {
      }
    }
    n170 = call "SeCrTs-Loop control.vi"("Action"=enum16{"Init", "Write", "Read"}."Read") -> ("Loop Control out"=w393:T14)  [unwired: 9 in, 1 out]
    n171 = call "SeCrTs-Error handler RT.vi"("error in"=w392, "Message Queue"=w390) -> ("error out"=w391:errorcluster)  [unwired: 8 in, 1 out]
    n172 = Unbundle By Name(w393) -> ("RT Stop"=w400:bool)
  }
  n173 = node-c288(w3) -> ()  [unwired: 1 out]
